vi "TTA_Grab_Fixture_Loss.vi"(1 "EXA VISA Resource":refnum<visa-resource-name>, 2 "MXG VISA Resource":refnum<visa-resource-name>) -> ()   [LabVIEW 2016]
panel:
  in  "error in":errorcluster
  in  "Frequency (MHz)":dbl
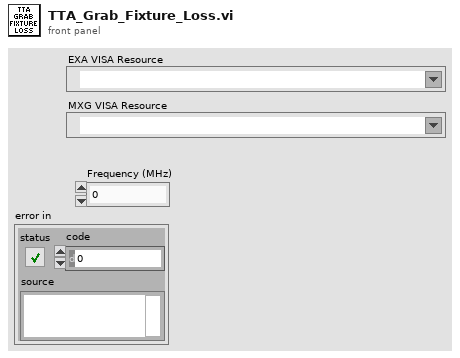
[diagram p1: front panel]
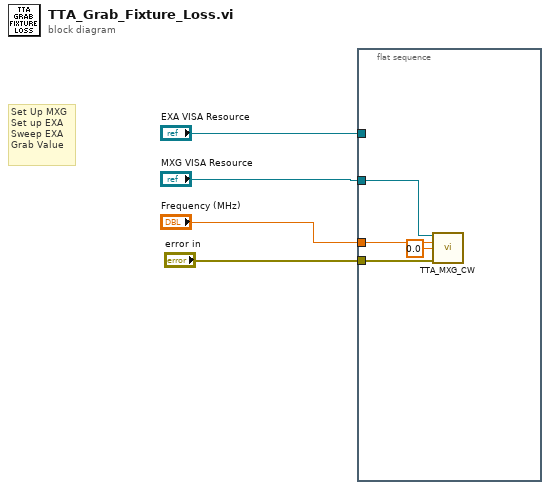
[diagram p0: block diagram]
diagram:
  # "Set Up MXG\nSet up EXA\nSweep EXA\nGrab Value"
  n1 = flat-sequence {
    tunnel: "EXA VISA Resource" -> [_]
    tunnel: "MXG VISA Resource" -> [w7]
    tunnel: "error in" -> [w8]
    tunnel: "Frequency (MHz)" -> [w6]
    frame #0 {
      n2 = call "TTA_MXG_CW.vi"("VISA resource In"=w7, "Frequency (MHz)"=w6, "Output Power\nLevel (dBm)"=0.0 ("Output Power\nLevel (dBm)"), "error in"=w8) -> ()  [unwired: 10 in, 2 out]
    }
  }
